vi "Preset Index Sol.vi"(8 "error in":errorcluster, 10 "CCW?":bool) -> (0 "error out":errorcluster)   [LabVIEW 2021]
uses:
  Global Variables/FPGA GV.vi
  <vilib>/Utility/error.llb/Error Cluster From Error Code.vi
  <vilib>/rvi/errors/niLvFpgaAdjustHostInterfaceError.vi
  <vilib>/rvi/interface/nirviReadWriteControl/nirviReadWriteControl.xnode
  <vilib>/rvi/interface/Simulation/niFpgaSimulationCallBeginRW.vi
  NiFpgaLv.dll
panel:
  out "Iterations":i32
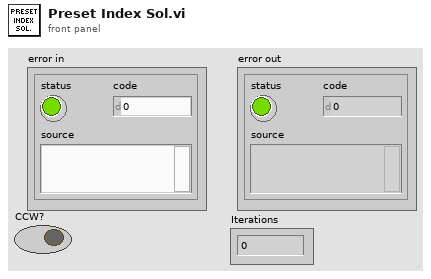
[diagram p1: front panel]
types:
  T1 = cluster{"TL_Red":bool, "TL_Orange":bool, "TL_Green":bool, "TL_Buzzer":bool, "Vaccuum ON":bool, "Vaccuum OFF":bool, "Beckhoff Data":bool, "SOL_Singling":bool, "Bowl Feeder_ ON1":bool, "Buffer 1":bool, "SOL_Pick_Place_Vertical":bool, "SOL_Tube_Feed_Agitatator":bool, "SOL_Tube_Feed_Gating_CYL":bool, "SOL_Insertion _CYL":bool, "SOL_Insertion_Clamp_CYL":bool, "SOL_Cutting_CYL":bool, "SOL_Cutting_Clamp_CYL":bool, "SOL_Insertion_Air_Nozzle":bool, "SOL_Measurement_CYL":bool, "SOL_Pick_Place_Rotary":bool, "SOL_Rejection CYL_1":bool, "SOL_Rejection CYL_2":bool, "SOL_Rejection CYL_3":bool, "SOL_Rejection CYL_4":bool, "Bowl Feeder_ON2":bool, "Linear Feeder 1":bool, "Linear Feeder 2":bool, "Buffer 2":bool, "Buffer 3":bool, "Buffer 4":bool, "Buffer 5":bool, "Buffer 6":bool}
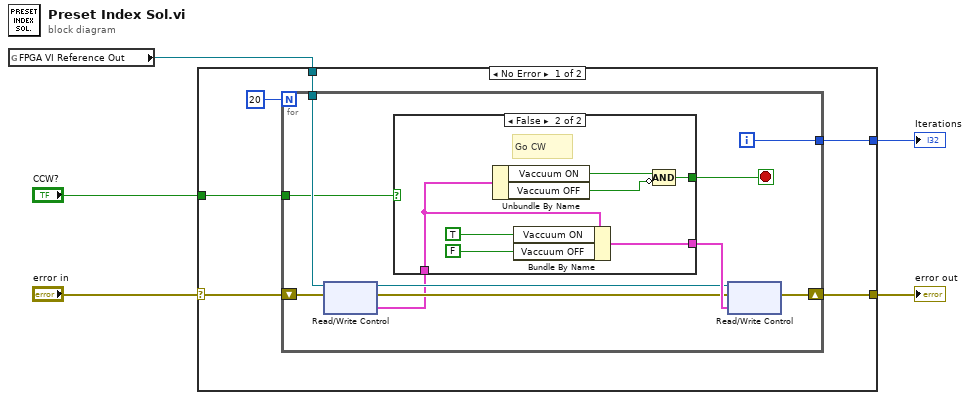
[diagram p0: block diagram]
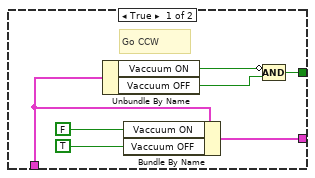
[diagram p2: hidden frame]
diagram:
  n1 = global read "FPGA GV.vi" "FPGA VI Reference Out"() -> (w3:refnum<k20>)
  n2 = case shown="No Error" "error in" {
    selector: "error in" -> [w10 w36]
    tunnel: [w11 w36] -> w5
    tunnel: w3 -> [w9 _]
    tunnel: "CCW?" -> [w7 _]
    tunnel: [w6 _] -> w1
    frame No Error {
      n3 = for {
        N: 20 -> [_]
        tunnel: w9 -> [w21]
        shift-right: [w16] -> w11
        shift-left: w10 -> [w17]
        tunnel: [w14] -> w6
        tunnel: w7 -> [w12]
        i -> [w14]
        stop <- w15 stop-if-true
        n4 = xnode "Read/Write Control"("FPGA VI Reference In"=w21, "error in"=w17) -> ("FPGA VI Reference Out"=w18:refnum<k20>, "error out"=w19:errorcluster, "DO 1"=w13:T1)
        n5 = case shown="False" w12 {
          tunnel: [w28 w35] -> w20
          tunnel: [w25 w32] -> w15
          tunnel: w13 -> [w22 w29]
          frame True {
            # "Go CCW"
            n6 = Unbundle By Name(w22) -> ("Vaccuum ON"=w27:bool, "Vaccuum OFF"=w23:bool)
            n7 = Bundle By Name(cluster=w22, "Vaccuum ON"=FALSE ("Pump_CNVR_Motor _ON"), "Vaccuum OFF"=TRUE ("SOL_Index_CNVR_Rotary_CCW")) -> (w28:T1)
            n8 = Compound Arithmetic op=AND(invert w27, w23) -> (w25:bool)
          }
          frame False {
            # "Go CW"
            n9 = Unbundle By Name(w29) -> ("Vaccuum ON"=w34:bool, "Vaccuum OFF"=w30:bool)
            n10 = Bundle By Name(cluster=w29, "Vaccuum ON"=TRUE ("Pump_CNVR_Motor _ON"), "Vaccuum OFF"=FALSE ("SOL_Index_CNVR_Rotary_CCW")) -> (w35:T1)
            n11 = Compound Arithmetic op=AND(w34, invert w30) -> (w32:bool)
          }
        }
        n12 = xnode "Read/Write Control"("FPGA VI Reference In"=w18, "error in"=w19, "DO 1"=w20) -> ("error out"=w16:errorcluster)  [unwired: 1 out]
      }
    }
    frame Error {
    }
  }
  "error out" <- w5
  "Iterations" <- w1
